vi "Actor Template-Core_Initialize.vi"(0 "DD Actor Template-Core In":refnum<class "DD Actor Template-Core.lvclass">, 5 "Initialization Sequence":string, 7 "FTW Actor Instance Configuration":string, 11 "error in (no error)":errorcluster) -> (4 "DD Actor Template-Core Out":refnum<class "DD Actor Template-Core.lvclass">, 6 "Event Refnums":T1, 10 "Refresh Period":dbl, 15 "error out":errorcluster)   [LabVIEW 2015, in "DD Actor Template-Core.lvclass"]
uses:
  DD Actor Template-Core.lvclass
  source/actor/Message/Request/FTW-Message-IncomingRequest.lvclass
  source/actor/Message/Base/FTW-Message.lvclass
  DD Actor Template-Core.lvclass/DD Actor Template-Core.ctl
  source/JSON/core/FTW-JSON-Core-EncodingFlags.vi
  source/JSON/FTW-JSON-Parse.vi
  source/Reflection/FTW-Reflection-Type.vi
  source/CodeGen/JSON Deserialize/FTW-JSON-Core-GetFlattenedValue.vi
  source/CodeGen/JSON Deserialize/FTW-JSON-Deserialize.xnode
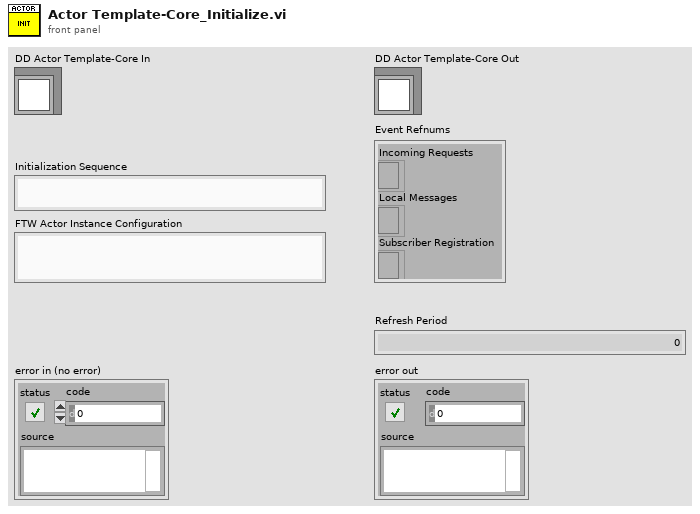
[diagram p1: front panel]
types:
  T1 = cluster{"Incoming Requests":refnum<event-registration>, "Local Messages":refnum<event-registration>, "Subscriber Registration":refnum<event-registration>}
  T2 = cluster{"My Data":bool, "Publisher URI":string, "Subscriber URIs":string, "Refresh Period":dbl}
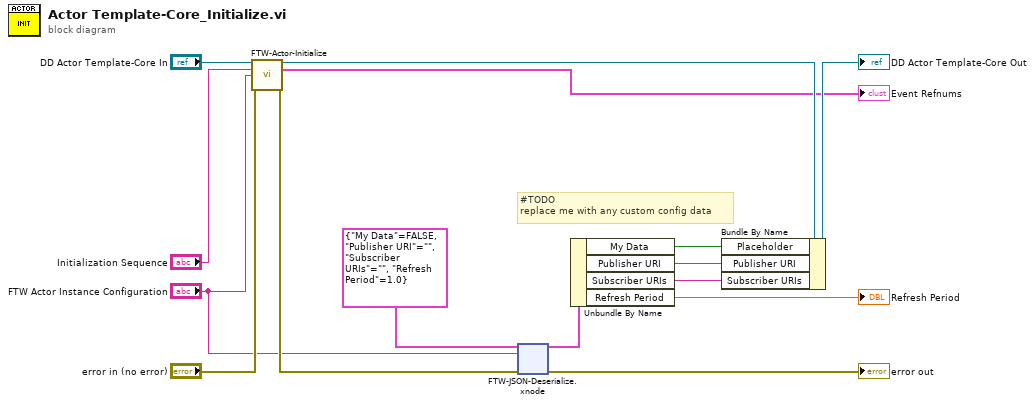
[diagram p0: block diagram]
diagram:
  # "#TODO\nreplace me with any custom config data"
  n1 = call-dynamic "FTW-Actor-Initialize.vi"("FTW Actor Instance Type"="DD Actor Template-Core In", "Initialization Job Sequence"="Initialization Sequence", "Actor Instance Configuration"="FTW Actor Instance Configuration", "error in"="error in (no error)") -> ("FTW Actor Instance"=w9:refnum<class "DD Actor Template-Core.lvclass">, "Event Refnums"=→"Event Refnums":T1, "error out"=w7:errorcluster)  [unwired: 9 in]
  n2 = xnode "FTW-JSON-Deserialize.xnode"("Type and Defaults"=T2 {"My Data"=FALSE, "Publisher URI"="", "Subscriber URIs"="", "Refresh Period"=1.0}, "JSON String"="FTW Actor Instance Configuration", "error in"=w7) -> ("Values"=w11:T2, "error out"=→"error out":errorcluster)
  n3 = Unbundle By Name(w11) -> ("My Data"=w10:bool, "Publisher URI"=w3:string, "Subscriber URIs"=w2:string, "Refresh Period"=→"Refresh Period":dbl)
  n4 = Bundle By Name(cluster=w9, "Placeholder"=w10, "Publisher URI"=w3, "Subscriber URIs"=w2) -> (→"DD Actor Template-Core Out":refnum<class "DD Actor Template-Core.lvclass">)
